vi "[TN#5] Measuring Complete Example(A).vi"() -> ()   [LabVIEW 2012]
uses:
  C:/Program Files/Metrohm Autolab/Autolab SDK 1.10/EcoChemie.Autolab.Sdk.dll
  EcoChemie.Autolab.Sdk.dll
panel:
  in  "Abort":bool
  in  "Save data as .nox (Path + filename.nox)":string
  out "Measurement active":bool
  in  "Save":bool
  in  "start measure":bool
  out "Y axis value":dbl
  out "X axis value":dbl
  out "Measured data":cluster{"Y":dbl[], "Y":dbl[]}[](graph)
  in  "X axis Signal":string(combo)
  in  "Y axis Signal":string(combo)
  in  "Embedded Exe File":path
  out "Blacklisted Commands detected":bool
  out "0, 1":i16
  in  "BoolSet":bool
  out "EnumGet":i32(ring) items=["Off", "On"]
  in  "SetEnum":bool
  in  "EnumSet":i32(ring) items=["Off", "On"]
  in  "Command name":string(combo)
  in  "Command parameter":string(combo)
  out "DoubleGet":dbl
  out "IntGet":i32
  in  "DoubleSet":dbl
  in  "IntSet":i32
  in  "SetBool":bool
  in  "SetDouble":bool
  in  "SetInt":bool
  in  "GetSet Parameter":bool
  in  "Hardware Setup File":path
  in  "Load":bool
  in  "data":bool
  in  "Stop":bool
  in  "Y axis signal":string(combo)
  in  "X axis signal":string(combo)
  in  "Procedure Command name":string(combo)
  out "Measured data":cluster{"Values":dbl[], "Values":dbl[]}(graph)
  in  "Load Procedure":path
  out "Autolab Connected":bool
  # "Edit parameter"
  # "Current parameter"
  # "Real-time data"
  # "Display Settings"
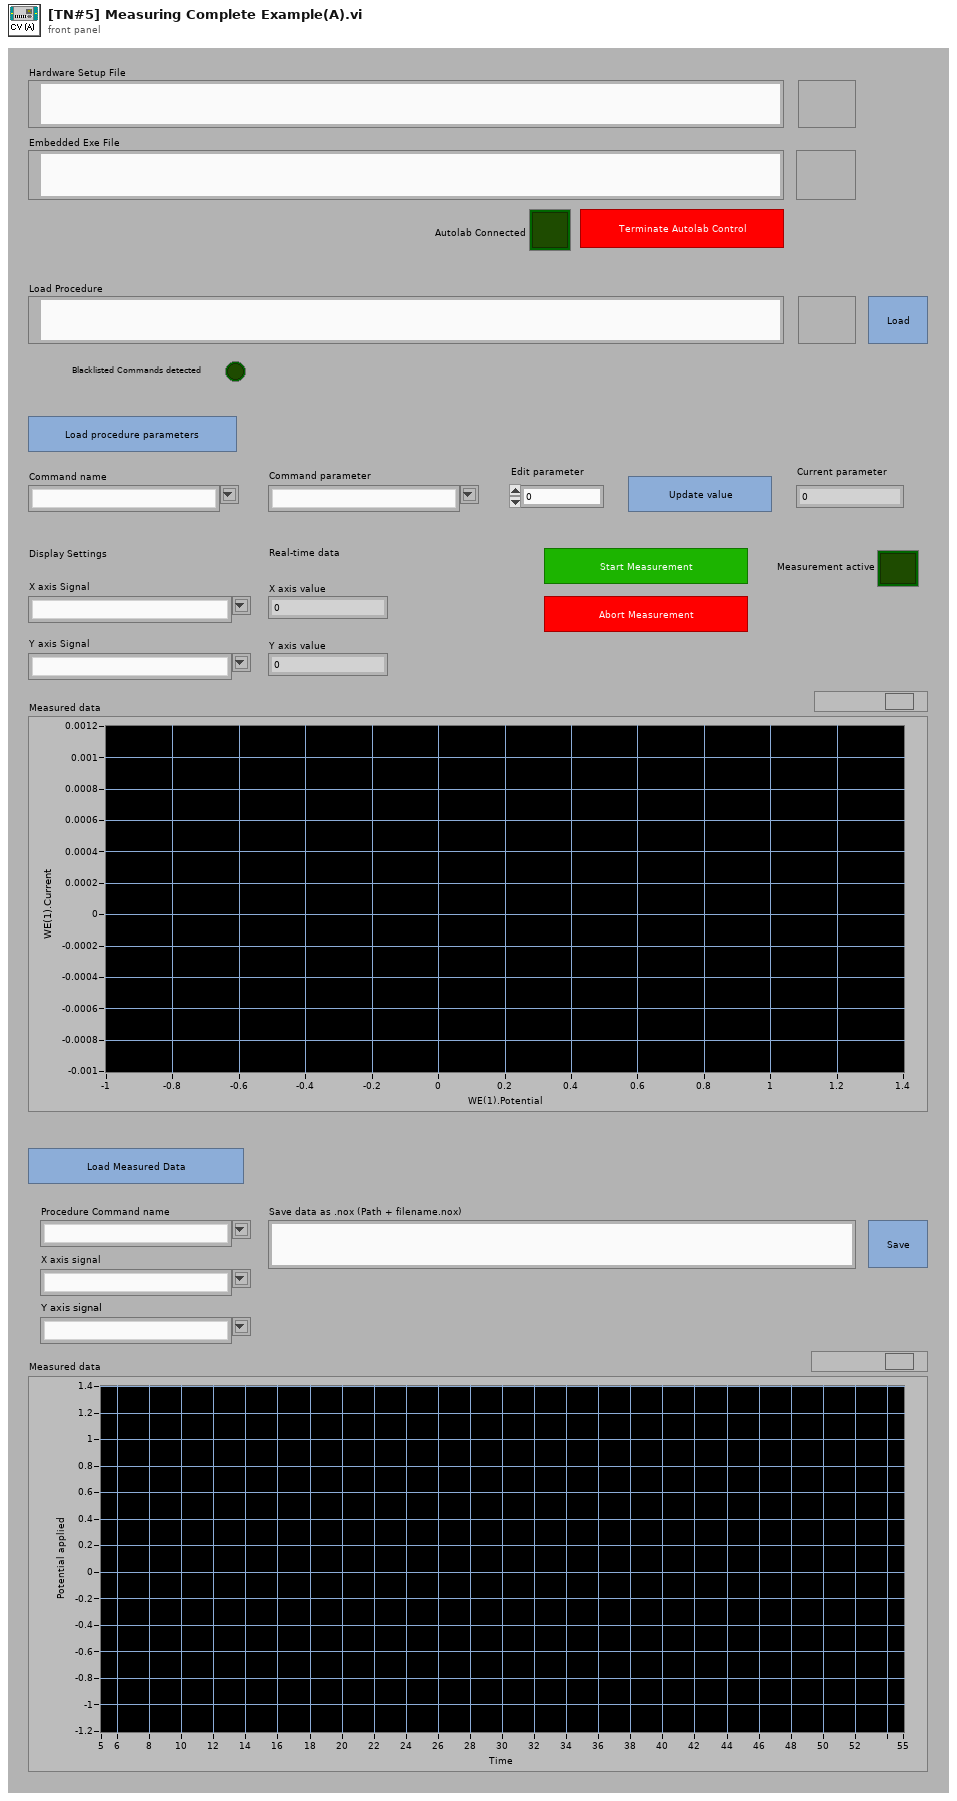
[diagram p1: front panel]
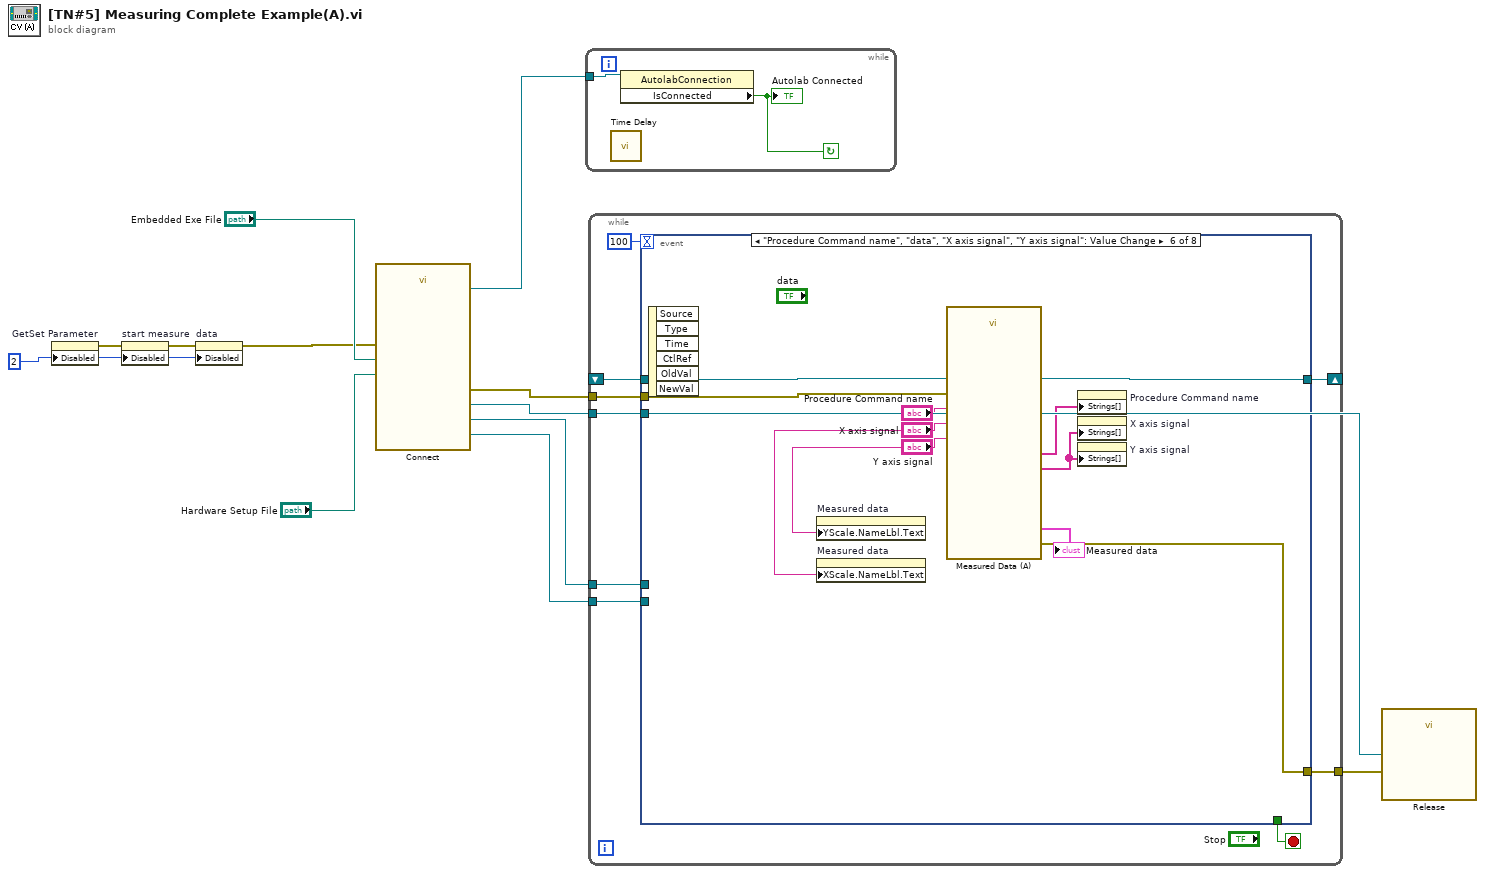
[diagram p0: block diagram]
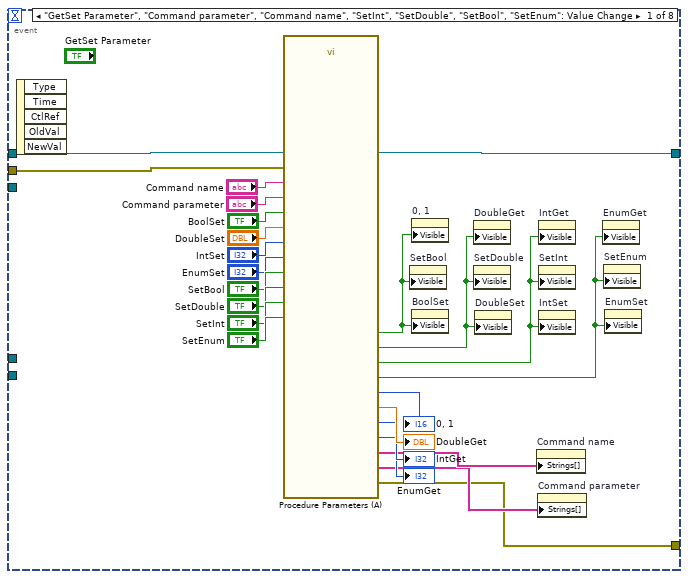
[diagram p2: hidden frame]
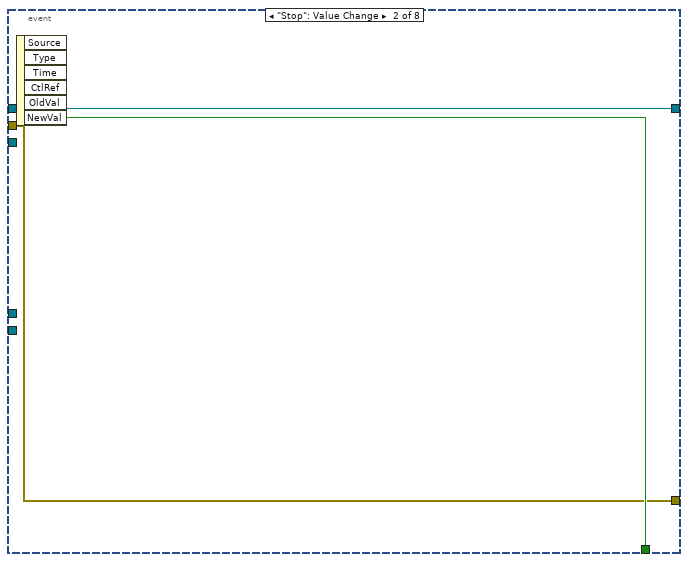
[diagram p3: hidden frame]
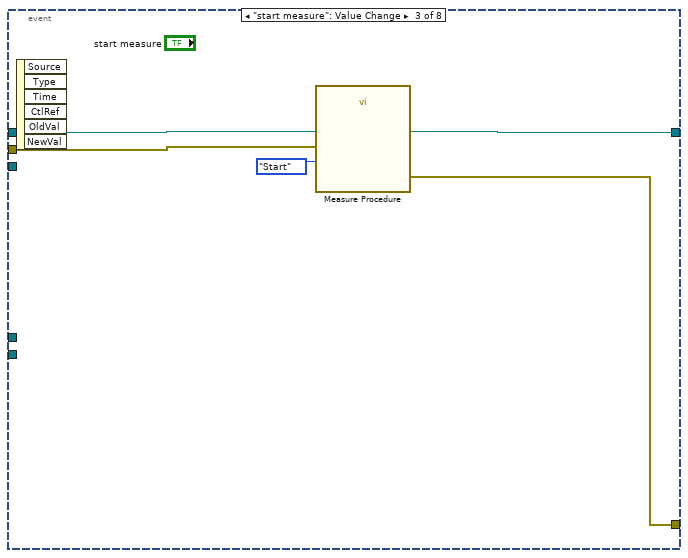
[diagram p4: hidden frame]
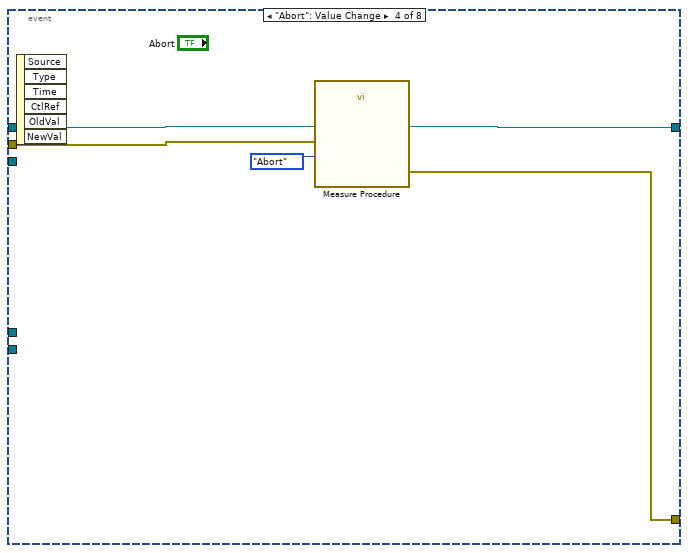
[diagram p5: hidden frame]
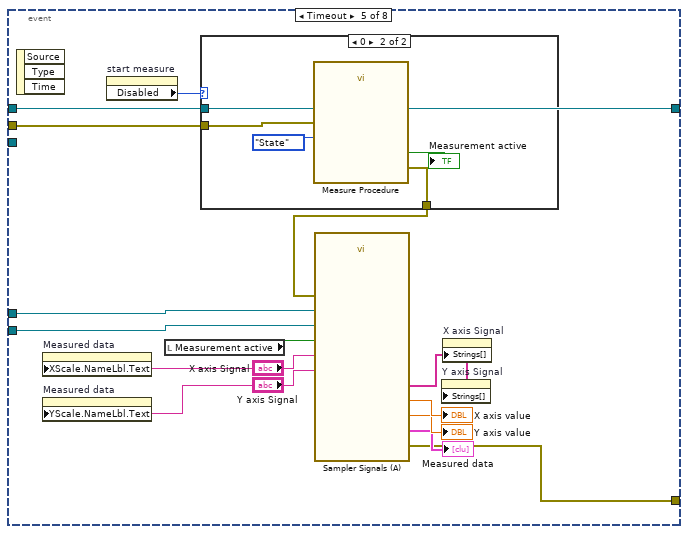
[diagram p6: hidden frame]
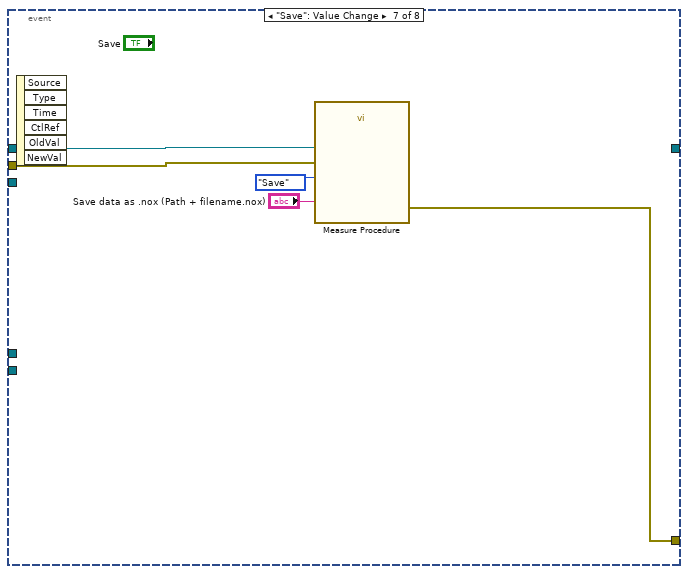
[diagram p8: hidden frame]
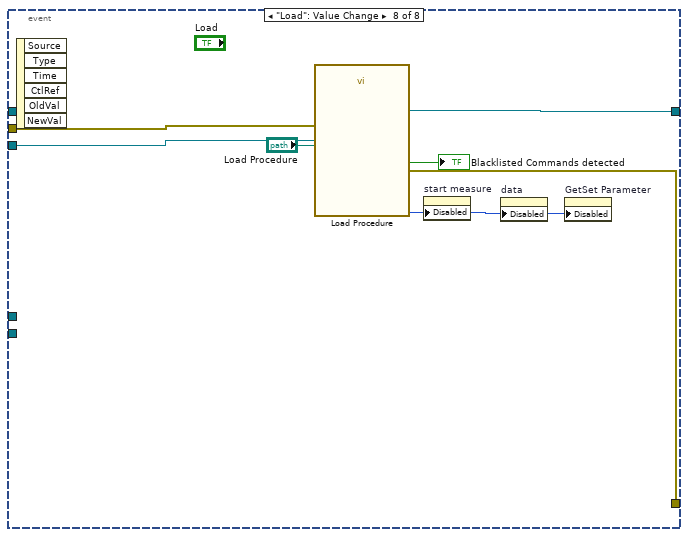
[diagram p9: hidden frame]
diagram:
  w8 = u8 2 ("Disabled")
  n1 = property on="GetSet Parameter" class="Bool (strict)"("Disabled"=w8) -> (error out=w7:errorcluster)  [unwired: 2 in, 1 out]
  n2 = property on="start measure" class="Bool"(error in=w7, "Disabled"=w8) -> (error out=w6:errorcluster)  [unwired: 1 in, 1 out]
  n3 = property on="data" class="Bool"(error in=w6, "Disabled"=w8) -> (error out=w5:errorcluster)  [unwired: 1 in, 1 out]
  n4 = call "Connect.vi"("Embedded Exe File"="Embedded Exe File", "Hardware Setup File"="Hardware Setup File", "error in (no error)"=w5) -> ("Sampler"=w2:refnum<k24>, "AutolabConnection"=w12:refnum<k24>, "instrument"=w3:refnum<k24>, "Ei"=w1:refnum<k24>, "error out"=w4:errorcluster)  [unwired: 8 out]
  n5 = while {
    tunnel: w12 -> [w13]
    stop <- w14 continue-if-true
    n6 = call "Time Delay"() -> ()  [unwired: 2 in, 10 out]
    n7 = property class="AutolabConnection"(reference=w13) -> ("IsConnected"=w14:bool)  [unwired: 1 in, 2 out]
    "Autolab Connected" <- w14
  }
  n8 = while {
    tunnel: [w21] -> w9
    shift-right: [w20] -> _
    shift-left: _ -> [w17]
    tunnel: w4 -> [w19]
    tunnel: w3 -> [w18]
    tunnel: w2 -> [w16]
    tunnel: w1 -> [w15]
    stop <- w22 stop-if-true
    n9 = event shown="[5] \"Procedure Command name\", \"data\", \"X axis signal\", \"Y axis signal\": Value Change" {
      selector: _ -> [_ _ _ _ _ _ _ _]
      dyn-events: _ -> [_ _ _ _ _ _ _ _]
      timeout: 100 -> [_ _ _ _ _ _ _ _]
      tunnel: [_ w49 _ _ _ _ _ _] -> w22
      tunnel: [w26 w48 w51 w55 w61 w78 w87 w92] -> w21
      tunnel: [w24 w47 w52 w54 w60 w80 _ w95] -> w20
      tunnel: w19 -> [w25 w48 w50 w56 w65 w79 w88 w94]
      tunnel: w18 -> [_ _ _ _ _ _ _ w93]
      tunnel: w17 -> [w24 w47 w52 w54 w60 w80 w89 _]
      tunnel: w16 -> [_ _ _ _ w63 _ _ _]
      tunnel: w15 -> [_ _ _ _ w62 _ _ _]
      event "GetSet Parameter", "Command parameter", "Command name", "SetInt", "SetDouble", "SetBool", "SetEnum": Value Change {
        n10 = event-data() -> ()  [unwired: 6 out]
        n11 = call "Procedure Parameters (A).vi"("LoadProcedure"=w24, "Command"="Command name", "Command Parameter"="Command parameter", "EnumSet"="EnumSet", "DoubleSet"="DoubleSet", "IntSet"="IntSet", "BoolSet"="BoolSet", "SetEnum"="SetEnum", "SetDouble"="SetDouble", "SetInt"="SetInt", "SetBool"="SetBool", "error in (no error)"=w25) -> ("error out"=w26:errorcluster, "IntGet"=→"IntGet":i32, "0, 1"=→"0, 1":i16, "EnumGet"=→"EnumGet":i32, "DoubleGet"=→"DoubleGet":dbl, "Command Names"=w28:string[], "Command Parameters"=w27:string[], "VisibleEnum"=w33:bool, "VisibleInt"=w34:bool, "VisibleDouble"=w35:bool, "VisableBool"=w36:bool)  [unwired: 1 in, 4 out]
        n12 = property on="SetBool" class="Bool (strict)"("Visible"=w36) -> ()  [unwired: 2 in, 2 out]
        n13 = property on="0, 1" class="DigNum (strict)"("Visible"=w36) -> ()  [unwired: 2 in, 2 out]
        n14 = property on="BoolSet" class="Bool (strict)"("Visible"=w36) -> ()  [unwired: 2 in, 2 out]
        n15 = property on="DoubleGet" class="DigNum (strict)"("Visible"=w35) -> ()  [unwired: 2 in, 2 out]
        n16 = property on="SetDouble" class="Bool (strict)"("Visible"=w35) -> ()  [unwired: 2 in, 2 out]
        n17 = property on="DoubleSet" class="DigNum (strict)"("Visible"=w35) -> ()  [unwired: 2 in, 2 out]
        n18 = property on="Command name" class="CmbBox"("Strings[]"=w28) -> ()  [unwired: 2 in, 2 out]
        n19 = property on="Command parameter" class="CmbBox"("Strings[]"=w27) -> ()  [unwired: 2 in, 2 out]
        n20 = property on="IntGet" class="DigNum (strict)"("Visible"=w34) -> ()  [unwired: 2 in, 2 out]
        n21 = property on="SetInt" class="Bool (strict)"("Visible"=w34) -> ()  [unwired: 2 in, 2 out]
        n22 = property on="IntSet" class="DigNum (strict)"("Visible"=w34) -> ()  [unwired: 2 in, 2 out]
        n23 = property on="EnumGet" class="Ring (strict)"("Visible"=w33) -> ()  [unwired: 2 in, 2 out]
        n24 = property on="SetEnum" class="Bool (strict)"("Visible"=w33) -> ()  [unwired: 2 in, 2 out]
        n25 = property on="EnumSet" class="Ring (strict)"("Visible"=w33) -> ()  [unwired: 2 in, 2 out]
      }
      event "Stop": Value Change {
        n26 = event-data() -> ("NewVal"=w49:bool)  [unwired: 6 out]
      }
      event "start measure": Value Change {
        n27 = event-data() -> ()  [unwired: 7 out]
        n28 = call "Measure Procedure.vi"("error in"=w50, "Request for procedure"=enum16{"State", "Save", "Abort", "Start"}."Start", "LoadProcedure"=w52) -> ("error out"=w51:errorcluster)  [unwired: 1 in, 7 out]
      }
      event "Abort": Value Change {
        n29 = event-data() -> ()  [unwired: 7 out]
        n30 = call "Measure Procedure.vi"("error in"=w56, "Request for procedure"=enum16{"State", "Save", "Abort", "Start"}."Abort", "LoadProcedure"=w54) -> ("error out"=w55:errorcluster)  [unwired: 1 in, 7 out]
      }
      event Timeout {
        n31 = event-data() -> ()  [unwired: 4 out]
        n32 = property on="Measured data" class="XYGraph (strict)"("XScale.NameLbl.Text"="X axis Signal") -> ()  [unwired: 2 in, 2 out]
        n33 = property on="Measured data" class="XYGraph (strict)"("YScale.NameLbl.Text"="Y axis Signal") -> ()  [unwired: 2 in, 2 out]
        n34 = property on="start measure" class="Bool"() -> ("Disabled"=w59:u8)  [unwired: 2 in, 2 out]
        n35 = local read "Measurement active"() -> (w58:bool)
        n36 = case shown="0" w59 {
          tunnel: w60 -> [_ w76]
          tunnel: w65 -> [w72 w75]
          tunnel: [w72 w74] -> w64
          frame 2, Default {
          }
          frame 0 {
            n37 = call "Measure Procedure.vi"("error in"=w75, "Request for procedure"=enum16{"State", "Save", "Abort", "Start"}."State", "LoadProcedure"=w76) -> ("error out"=w74:errorcluster, "IsMeasuring"=→"Measurement active":bool)  [unwired: 1 in, 6 out]
          }
        }
        n38 = call "Sampler Signals (A).vi"("IsMeasuring"=w58, "EI"=w62, "Sampler"=w63, "Signal X"="X axis Signal", "Signal Y"="Y axis Signal", "error in"=w64) -> ("X"=→"X axis value":dbl, "Y"=→"Y axis value":dbl, "XY Graph"=→"Measured data":cluster{"Y":dbl[], "Y":dbl[]}[], "GetSignals"=w69:string[], "error out"=w61:errorcluster)  [unwired: 4 in, 1 out]
        n39 = property on="Y axis Signal" class="CmbBox"("Strings[]"=w69) -> ()  [unwired: 2 in, 2 out]
        n40 = property on="X axis Signal" class="CmbBox"("Strings[]"=w69) -> ()  [unwired: 2 in, 2 out]
      }
      event "Procedure Command name", "data", "X axis signal", "Y axis signal": Value Change {
        n41 = event-data() -> ()  [unwired: 7 out]
        n42 = property on="Measured data" class="XYGraph (strict)"("YScale.NameLbl.Text"="Y axis signal") -> ()  [unwired: 2 in, 2 out]
        n43 = property on="Measured data" class="XYGraph (strict)"("XScale.NameLbl.Text"="X axis signal") -> ()  [unwired: 2 in, 2 out]
        n44 = call "Measured Data (A).vi"("LoadProcedure"=w80, "ProcedureCommandList"="Procedure Command name", "Signal X sel"="X axis signal", "Signal Y sel"="Y axis signal", "error in (no error)"=w79) -> ("Signal Names"=w83:string[], "ProcedureCommandList"=w82:string[], "XY Graph"=→"Measured data":cluster{"Values":dbl[], "Values":dbl[]}, "error out"=w78:errorcluster)  [unwired: 7 out]
        n45 = property on="Procedure Command name" class="CmbBox"("Strings[]"=w82) -> ()  [unwired: 2 in, 2 out]
        n46 = property on="X axis signal" class="CmbBox"("Strings[]"=w83) -> ()  [unwired: 2 in, 2 out]
        n47 = property on="Y axis signal" class="CmbBox"("Strings[]"=w83) -> ()  [unwired: 2 in, 2 out]
      }
      event "Save": Value Change {
        n48 = event-data() -> ()  [unwired: 7 out]
        n49 = call "Measure Procedure.vi"("error in"=w88, "fileName"="Save data as .nox (Path + filename.nox)", "Request for procedure"=enum16{"State", "Save", "Abort", "Start"}."Save", "LoadProcedure"=w89) -> ("error out"=w87:errorcluster)  [unwired: 7 out]
      }
      event "Load": Value Change {
        n50 = event-data() -> ()  [unwired: 7 out]
        n51 = call "Load Procedure.vi"("error in (no error)"=w94, "Procedure"="Load Procedure", "Instrument"=w93) -> ("error out"=w92:errorcluster, "Contains"=→"Blacklisted Commands detected":bool, "Numeric"=w96:i32, "LoadProcedure"=w95:refnum<k24>)  [unwired: 5 out]
        n52 = property on="start measure" class="Bool"("Disabled"=w96) -> ()  [unwired: 2 in, 2 out]
        n53 = property on="data" class="Bool"("Disabled"=w96) -> ()  [unwired: 2 in, 2 out]
        n54 = property on="GetSet Parameter" class="Bool (strict)"("Disabled"=w96) -> ()  [unwired: 2 in, 2 out]
      }
    }
  }
  n55 = call "Release.vi"("error in (no error)"=w9, "Instrument"=w3) -> ()  [unwired: 1 in, 9 out]
